vi "CheckOverload.vi"() -> (0 "Error Out":errorcluster)   [LabVIEW 2015]
doc: "Configures device parameters for an NI 5170/5171"
uses:
  OscopeAPI/Device Session.lvclass
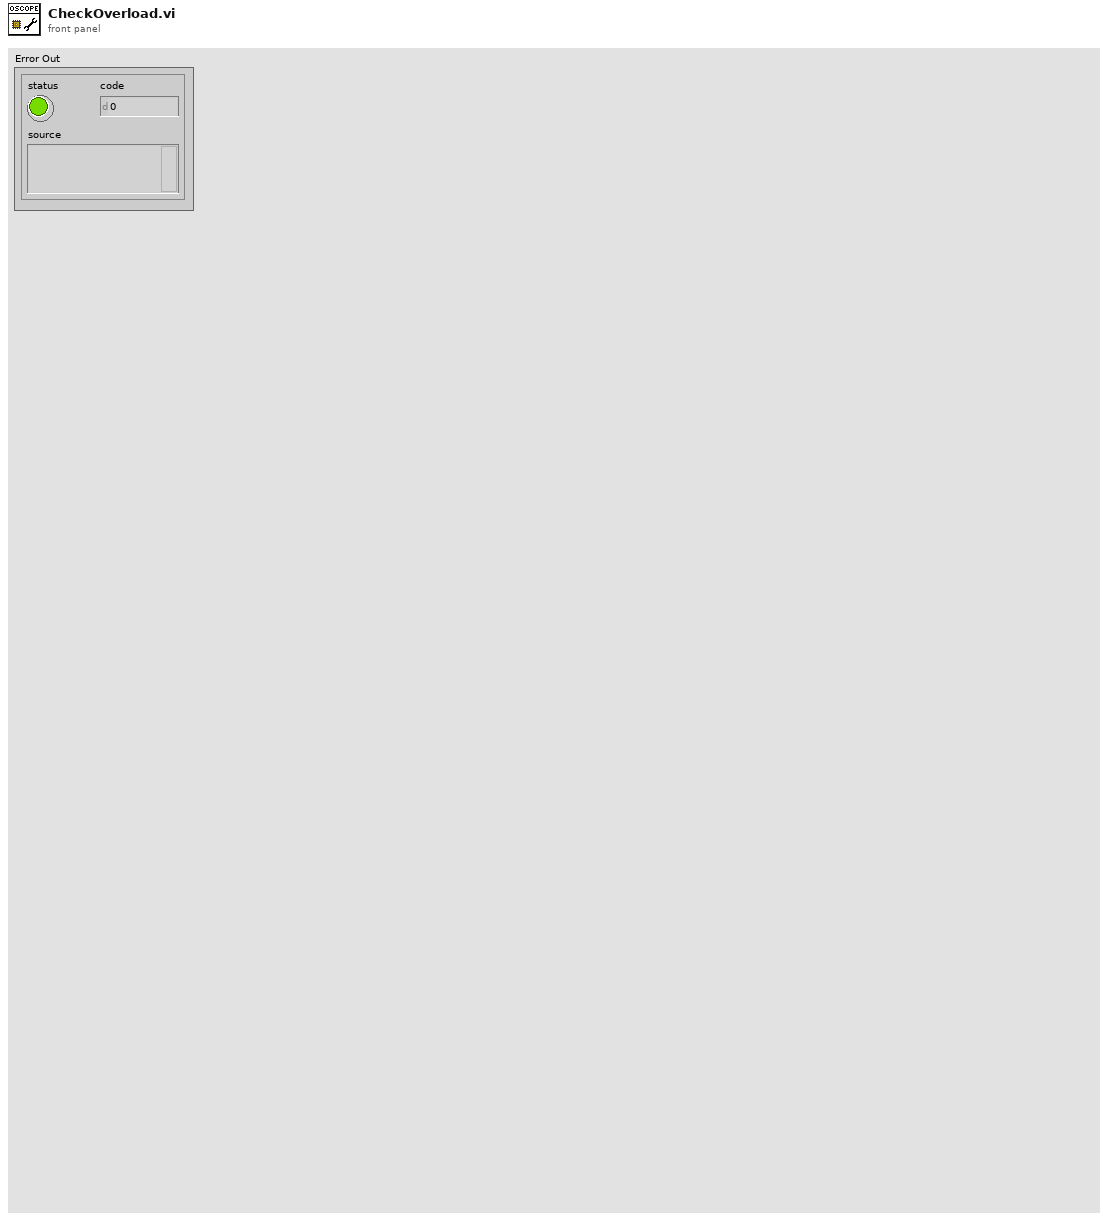
[diagram p1: front panel]
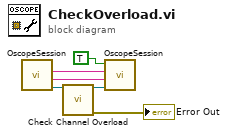
[diagram p0: block diagram]
diagram:
  n1 = call "OscopeSession.vi"() -> ("Session Out"=w3:refnum<class "Device Session.lvclass">, "Bitfile Path Out"=w1:string, "Device Address Out"=w2:string)  [unwired: 9 in]
  n2 = call "Check Channel Overload.vi"("device session in"=w3) -> ("device session out"=w5:refnum<class "Device Session.lvclass">, "error out"=→"Error Out":errorcluster)  [unwired: 13 in]
  n3 = call "OscopeSession.vi"("Session In"=w5, "Bitfile Path In"=w1, "Device Address In"=w2, "Write"=TRUE) -> ()  [unwired: 5 in, 3 out]
